vi "RVHR - Configure Language Settings.vi"(7 "Directory Path":path, 8 "error in (no error)":errorcluster, 10 "Supervisory Config Cluster Out":T2={"UI Information"={"Header Image"=path "../Data/header.png", "Language"=enum."English", "First Run?"=FALSE, "Setup Camera?"=FALSE, "Device Type"=enum."RCA", "Encoder Type"=enum."Tacho", "Version"=enum."RailMeasurement_CAT", "port"=0, "greyscale"=FALSE, "camera index"=0}, "Test Cluster"={"Operator"="", "Description"="", "Line"="", "Start Position"=450000.0, "Run Length"=31.0, "Sensor A Position"=80000.0, "Rail Side"=FALSE, "Distance Direction"=FALSE, "Path"=path "", "Sensor B Position"=0.0, "Visible Chart Distance"=0.0, "Company"="", "Ref Profile"=""}, "RV-HR Settings Cluster"={"Sensor A Calibration"=0.0, "Integrator Time"=0.0, "Encoder Spacing"=0.0, "Encoder Threshold"=0.0, "Sampling Distance"=0, "Swap Direction?"=FALSE, "Min Walking Speed"=0.0, "Max Walking Speed"=0.0, "Distance Format"=0, "Sensor B Calibration"=0.0, "Tacho Pulses/Rev"=0.0, "Wheel Diameter"=0.0, "Max Short Roughness"=0.0, "Max Long Roughness"=0.0, "Measuring Interval"=0.0, "Measuring Length"=0.0, "Wavelengths"=[], "Device Resolution"=0, "Detect Change in Direction?"=FALSE, "Save Images?"=FALSE, "Image Frequency"=0, "Save Video?"=FALSE, "Image Offset"=0.0, "Start Position at 0m?"=FALSE, "Live Corrug Est.?"=FALSE, "Wavelength Corrug"=0, "Distance Corrug"=0, "Update Corrug"=0}} {"RV-HR Settings Cluster"."Image Frequency" items=["2", "3", "5"]; "RV-HR Settings Cluster"."Device Resolution" items=["0.1 µm", "1 µm", "10 µm"]; "RV-HR Settings Cluster"."Distance Format" items=["kilometres", "miles & chains", "metres", "stations", "miles"]; "RV-HR Settings Cluster"."Sampling Distance" items=["1mm", "2mm"]}, 11 "UI References":T13) -> (0 "error out":errorcluster, 2 "Language Config Cluster Out":T1={"Home"="Home", "Test Setup"="Setup", "Run Test"="Test", "Configure"="Config", "Hardware Viewer"="Viewer", "Review Test"="Review", "Report"="Home", "Exit"="Exit", "Device Connected?"="Device Connected?", "Test in Progress?"="Test in Progress?", "Simulate?"="Simulate?", "Device Type 1"="Corrugation Analysis Trolley", "Device Type 2"="Bi-Corrugation Analysis Trolley", "Device Type 3"="Bi-Corrugation Analysis Trolley", "Device Type 4"="Bi-Corrugation Analysis Trolley", "Device Type 5"="Bi-Corrugation Analysis Trolley", "Device Type 6"="Bi-Corrugation Analysis Trolley", "Device Type 7"="Bi-Corrugation Analysis Trolley", "Software Version"="Version", "Support"="Software by RailMeasurement Limited - Cambridge - UK - support@railmeasurement.com", "Operator"="Operator:", "Test Description"="Description:", "Line"="Description:", "Test Folder Path"="Folder Path:", "Test Folder Path RCA"="Folder Path:", "Start Position"="Start Position:", "Sensor Position"="Sensor Position:", "Sensor A Position"="Sensor A Position:", "Sensor B Position"="Sensor B Position:", "Visible Chart Distance"="Sensor B Position:", "Rail Side"="Rail Side:", "Rail A Side"="Rail A Side:", "Distance Direction"="Distance Direction:", "Start"="Start:", "Distance Travelled"="Distance Travelled:", "Current Position"="Current Position:", "Stop Test"="Stop", "Pause Test"="Save", "Displacement"="Displacement", "Position"="Position", "Sensor Calibration"="Sensor Calibration:", "Sensor A Calibration"="Sensor A Calibration:", "Sensor B Calibration"="Sensor B Calibration:", "Encoder Spacing"="Encoder Spacing:", "Sampling Distance"="Sampling Distance:", "Tacho Pulses/Rev"="Sensor Calibration:", "Wheel Diameter"="Sensor A Calibration:", "Sampling Distances"=["1mm", "2mm"], "Distance Unit"="Distance in:", "Distance Units"=["Kilometres", "miles & chains", "metres", "stations", "miles"], "Swap Direction"="Swap Direction at Run End?", "Language"="Language", "Device Resolution"="Save", "Device Resolutions"=["Kilometres", "miles & chains", "metres", "stations", "miles"], "Detect Change in Direction"="Save", "Save Config"="Save", "Encoder Data"="Encoder Data", "Sensor Data"="Sensor Data", "Sensor A Data"="Sensor A Data", "Sensor B Data"="Sensor B Data", "Voltage"="Voltage", "Time (m:s)"="Time (m:s)", "Unit mm/s/V"="(mm/s)/V", "Unit mm"="mm", "Unit km"="km", "Unit m"="m", "Start Test Message"="m", "Stop Test Message"="km", "Exit Message"="mm", "File Exists Message"="mm", "File Path Invalid Message"="mm", "Combine Error"="mm", "Combine Success"="mm", "Roller Comp Error"="mm", "Test Folder Path (Live)"="mm", "Folder Error"="Sensor B Position:", "Enc Count"="Setup", "Run Start"="mm", "Run End"="mm", "Date"="mm", "Train"="Sensor B Position:", "Location"="Setup", "Notes"="mm", "Heading_1"="mm", "Heading_2"="mm", "Left Rail"="Sensor B Position:", "Right Rail"="Setup", "Left Exclusions"="mm", "Right Exclusions"="mm", "Settings"="mm", "Wavelength Ranges"="Sensor B Position:", "Y-Axis Limits"="Setup", "Exc Limits"="Sensor B Position:", "Other Settings"="Setup", "Distance/Page"="mm", "Distance/Pages"=["Kilometres", "miles & chains", "metres", "stations", "miles"], "Gridlines"="mm", "Report Tolerance"="mm", "Manual Cut"="Sensor B Position:", "Plot Colour"="Distance in:", "Plot Colours"=["Kilometres", "miles & chains", "metres", "stations", "miles"], "EN Standard"="mm", "RiL Standard"="mm", "Custom Standard"="mm", "Resolution"="Distance in:", "Resolutions"=["Kilometres", "miles & chains", "metres", "stations", "miles"], "Exceedence Header"="mm", "Distance (km)"="mm", "Left (%)"="mm", "Right (%)"="Distance in:", "Page"="Distance in:", "Align"="mm", "Main"="mm", "Comparison"="Distance in:", "Offset"="Distance in:", "From"="Distance in:", "To"="Distance in:", "Of"="Distance in:", "File"="mm", "Load New"="mm", "Load Comparison"="Distance in:", "Discard Comparison"="Distance in:", "Print Current Page"="Distance in:", "Print All Pages"="Distance in:", "Print Exceedence Report"="Distance in:", "Plot Main"="Distance in:", "No Comparison Data to Align"="Distance in:", "Run Load Error"="Distance in:", "Report Load Error"="Distance in:", "Cut"="Distance in:", "Remove"="Distance in:", "Config Settings Unsaved"="Distance in:", "Acquisition Paused"="Distance in:", "Please Select One Option Below"="Distance in:", "RCA is Now Stationary"="Distance in:", "Reporting Setting"="Distance in:", "Main Abbreviated"="Distance in:", "Comparison Abbreviated"="Distance in:", "Exceedence Abbreviated"="Distance in:", "Align Comparison"="Distance in:", "Rail Corrugation Analyser Reporting"="Distance in:", "Show Exc. % in Graph"="Distance in:", "Evaluate Sections <100m"="Distance in:", "Evaluate Sections <0.062mile"="Distance in:", "Section Too Short for Evaluation"="Distance in:", "Language Change Prompt"="Distance in:", "Show All"="Distance in:", "Sections_km"="Distance in:", "Sections_mi"="Distance in:", "Vision"="Distance in:", "Vision Report"="Distance in:", "Vision Display"="Distance in:", "Vision Displays"=["Kilometres", "miles & chains", "metres", "stations", "miles"], "Save Images"="Distance in:", "Image Frequency"="Distance in:", "Section"="Distance in:", "Brightness"="Distance in:", "Contrast"="Distance in:", "Shadow"="Distance in:", "Sharpened"="Distance in:", "Apply to all Images"="Distance in:", "Reset"="Distance in:", "Are you sure"="Distance in:", "Image Processing"="Distance in:", "Save Video"="Distance in:", "Image Offset"="Distance in:", "Camera Mode"="Distance in:", "Camera Modes"=["Kilometres", "miles & chains", "metres", "stations", "miles"], "Copy Page"="Distance in:", "Copy Graphs"="Distance in:", "Camera Mode Change Prompt"="Distance in:", "Camera_1 Missing"="Distance in:", "Camera_2 Missing"="Distance in:", "Cameras Missing"="Distance in:", "Camera Setup"="Distance in:", "Camera_1 Connection Error"="Distance in:", "Camera_2 Connection Error"="Distance in:", "Cameras Connection Error"="Distance in:", "No GPS"="Distance in:", "No Signal"="Distance in:", "Camera_1 Connected"="Distance in:", "Camera_1 Not Connected"="Distance in:", "Camera_2 Connected"="Distance in:", "Camera_2 Not Connected"="Distance in:", "Start Position at 0m?"="Distance in:", "Continue"="Distance in:", "New Test, Same Direction"="Distance in:", "New Test, Opposite Direction"="Distance in:", "Stop and Save"="Distance in:", "Live Corrug Estimate"="Distance in:", "Wavelength Corrug"="Distance in:", "Distance Corrug "="Distance in:", "Update Corrug"="Distance in:", "Company"="Distance in:", "Ref Profile "="Distance in:"})   [LabVIEW 2024]
uses:
  Controls/RVHR - Setting refs.ctl
  Controls/Supervisory Config Cluster.ctl
  Controls/UI Init Config Info.ctl
  Controls/Language.ctl
  Controls/Device_Type.ctl
  Controls/EncoderType.ctl
  Controls/Software Version.ctl
  Controls/Test Cluster.ctl
  Controls/Settings Cluster.ctl
  Controls/Sampling DIstance.ctl
  Controls/Distance Units.ctl
  Controls/Device_Resolution.ctl
  Controls/Language Text Cluster.ctl
  <vilib>/addons/Tools/Unicode/UI Unicode Tools.lvlib
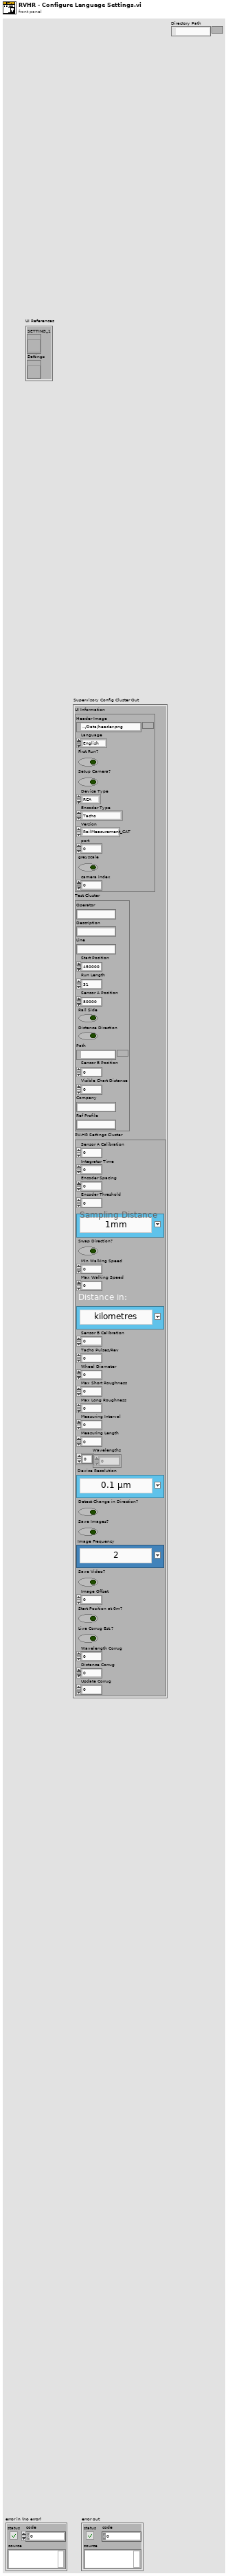
[diagram p1: front panel]
types:
  T1 = typedef "Language Text Cluster.ctl" = cluster{"Home":string, "Test Setup":string, "Run Test":string, "Configure":string, "Hardware Viewer":string, "Review Test":string, "Report":string, "Exit":string, "Device Connected?":string, "Test in Progress?":string, "Simulate?":string, "Device Type 1":string, "Device Type 2":string, "Device Type 3":string, "Device Type 4":string, "Device Type 5":string, "Device Type 6":string, "Device Type 7":string, "Software Version":string, "Support":string, "Operator":string, "Test Description":string, "Line":string, "Test Folder Path":string, "Test Folder Path RCA":string, "Start Position":string, "Sensor Position":string, "Sensor A Position":string, "Sensor B Position":string, "Visible Chart Distance":string, "Rail Side":string, "Rail A Side":string, "Distance Direction":string, "Start":string, "Distance Travelled":string, "Current Position":string, "Stop Test":string, "Pause Test":string, "Displacement":string, "Position":string, "Sensor Calibration":string, "Sensor A Calibration":string, "Sensor B Calibration":string, "Encoder Spacing":string, "Sampling Distance":string, "Tacho Pulses/Rev":string, "Wheel Diameter":string, "Sampling Distances":string[], "Distance Unit":string, "Distance Units":string[], "Swap Direction":string, "Language":string, "Device Resolution":string, "Device Resolutions":string[], "Detect Change in Direction":string, "Save Config":string, "Encoder Data":string, "Sensor Data":string, "Sensor A Data":string, "Sensor B Data":string, "Voltage":string, "Time (m:s)":string, "Unit mm/s/V":string, "Unit mm":string, "Unit km":string, "Unit m":string, "Start Test Message":string, "Stop Test Message":string, "Exit Message":string, "File Exists Message":string, "File Path Invalid Message":string, "Combine Error":string, "Combine Success":string, "Roller Comp Error":string, "Test Folder Path (Live)":string, "Folder Error":string, "Enc Count":string, "Run Start":string, "Run End":string, "Date":string, "Train":string, "Location":string, "Notes":string, "Heading_1":string, "Heading_2":string, "Left Rail":string, "Right Rail":string, "Left Exclusions":string, "Right Exclusions":string, "Settings":string, "Wavelength Ranges":string, "Y-Axis Limits":string, "Exc Limits":string, "Other Settings":string, "Distance/Page":string, "Distance/Pages":string[], "Gridlines":string, "Report Tolerance":string, "Manual Cut":string, "Plot Colour":string, "Plot Colours":string[], "EN Standard":string, "RiL Standard":string, "Custom Standard":string, "Resolution":string, "Resolutions":string[], "Exceedence Header":string, "Distance (km)":string, "Left (%)":string, "Right (%)":string, "Page":string, "Align":string, "Main":string, "Comparison":string, "Offset":string, "From":string, "To":string, "Of":string, "File":string, "Load New":string, "Load Comparison":string, "Discard Comparison":string, "Print Current Page":string, "Print All Pages":string, "Print Exceedence Report":string, "Plot Main":string, "No Comparison Data to Align":string, "Run Load Error":string, "Report Load Error":string, "Cut":string, "Remove":string, "Config Settings Unsaved":string, "Acquisition Paused":string, "Please Select One Option Below":string, "RCA is Now Stationary":string, "Reporting Setting":string, "Main Abbreviated":string, "Comparison Abbreviated":string, "Exceedence Abbreviated":string, "Align Comparison":string, "Rail Corrugation Analyser Reporting":string, "Show Exc. % in Graph":string, "Evaluate Sections <100m":string, "Evaluate Sections <0.062mile":string, "Section Too Short for Evaluation":string, "Language Change Prompt":string, "Show All":string, "Sections_km":string, "Sections_mi":string, "Vision":string, "Vision Report":string, "Vision Display":string, "Vision Displays":string[], "Save Images":string, "Image Frequency":string, "Section":string, "Brightness":string, "Contrast":string, "Shadow":string, "Sharpened":string, "Apply to all Images":string, "Reset":string, "Are you sure":string, "Image Processing":string, "Save Video":string, "Image Offset":string, "Camera Mode":string, "Camera Modes":string[], "Copy Page":string, "Copy Graphs":string, "Camera Mode Change Prompt":string, "Camera_1 Missing":string, "Camera_2 Missing":string, "Cameras Missing":string, "Camera Setup":string, "Camera_1 Connection Error":string, "Camera_2 Connection Error":string, "Cameras Connection Error":string, "No GPS":string, "No Signal":string, "Camera_1 Connected":string, "Camera_1 Not Connected":string, "Camera_2 Connected":string, "Camera_2 Not Connected":string, "Start Position at 0m?":string, "Continue":string, "New Test, Same Direction":string, "New Test, Opposite Direction":string, "Stop and Save":string, "Live Corrug Estimate":string, "Wavelength Corrug":string, "Distance Corrug ":string, "Update Corrug":string, "Company":string, "Ref Profile ":string}
  T2 = typedef "Supervisory Config Cluster.ctl" = cluster{"UI Information":T3, "Test Cluster":T8, "RV-HR Settings Cluster":T9}
  T3 = typedef "UI Init Config Info.ctl" = cluster{"Header Image":path, "Language":T4, "First Run?":bool, "Setup Camera?":bool, "Device Type":T5, "Encoder Type":T6, "Version":T7, "port":i32, "greyscale":bool, "camera index":i32}
  T4 = typedef "Language.ctl" = enum16{"English", "Chinese", "German"}
  T5 = typedef "Device_Type.ctl" = enum16{"CAT", "Bi-CAT", "YRCA", "RCA", "RV-HR", "TV-HR"}
  T6 = typedef "EncoderType.ctl" = enum16{"Tacho", "Quadrature"}
  T7 = typedef "Software Version.ctl" = enum16{"RailMeasurement_CAT", "RailMeasurement_Master", "RailMeasurement_RCA", "RailMeasurement_CAT-V", "RailMeasurement_RCA-V", "RailMeasurement_RV-HR"}
  T8 = typedef "Test Cluster.ctl" = cluster{"Operator":string, "Description":string, "Line":string, "Start Position":dbl, "Run Length":dbl, "Sensor A Position":dbl, "Rail Side":bool, "Distance Direction":bool, "Path":path, "Sensor B Position":dbl, "Visible Chart Distance":dbl, "Company":string, "Ref Profile":string}
  T9 = typedef "Settings Cluster.ctl" = cluster{"Sensor A Calibration":dbl, "Integrator Time":dbl, "Encoder Spacing":dbl, "Encoder Threshold":dbl, "Sampling Distance":T10, "Swap Direction?":bool, "Min Walking Speed":dbl, "Max Walking Speed":dbl, "Distance Format":T11, "Sensor B Calibration":dbl, "Tacho Pulses/Rev":dbl, "Wheel Diameter":dbl, "Max Short Roughness":dbl, "Max Long Roughness":dbl, "Measuring Interval":dbl, "Measuring Length":dbl, "Wavelengths":dbl[], "Device Resolution":T12, "Detect Change in Direction?":bool, "Save Images?":bool, "Image Frequency":T10, "Save Video?":bool, "Image Offset":dbl, "Start Position at 0m?":bool, "Live Corrug Est.?":bool, "Wavelength Corrug":u8, "Distance Corrug":u8, "Update Corrug":u8}
  T10 = typedef "Sampling DIstance.ctl" = u16
  T11 = typedef "Distance Units.ctl" = u16
  T12 = typedef "Device_Resolution.ctl" = u16
  T13 = typedef "RVHR - Setting refs.ctl" = cluster{"SETTING_1":refnum<vi>, "Settings":refnum<vi>}
  T14 = typedef "Settings UI Refs.ctl" = cluster{"10-30mm":refnum<vi>, "30-100mm":refnum<vi>, "100-300mm":refnum<vi>, "300-1000mm":refnum<vi>, "Y 10-30mm":refnum<vi>, "Y 30-100mm":refnum<vi>, "Y 100-300mm":refnum<vi>, "Y 300-1000mm":refnum<vi>, "Ex 10-30mm":refnum<vi>, "Ex 30-100mm":refnum<vi>, "Ex 100-300mm":refnum<vi>, "Ex 300-1000mm":refnum<vi>, "Exceedance Resolution":refnum<vi>, "EN13231?":refnum<vi>, "Ril?":refnum<vi>, "Custom?":refnum<vi>, "Distance Per Page":refnum<vi>, "Distance Per Page (Miles)":refnum<vi>, "Exc Limit":refnum<vi>, "Gridlines?":refnum<vi>, "Manual Cut?":refnum<vi>, "Plot Colours":refnum<vi>, "Wavelength Ranges":refnum<vi>, "Y-Axis Limits":refnum<vi>, "Exc Limits":refnum<vi>, "Settings":refnum<vi>}
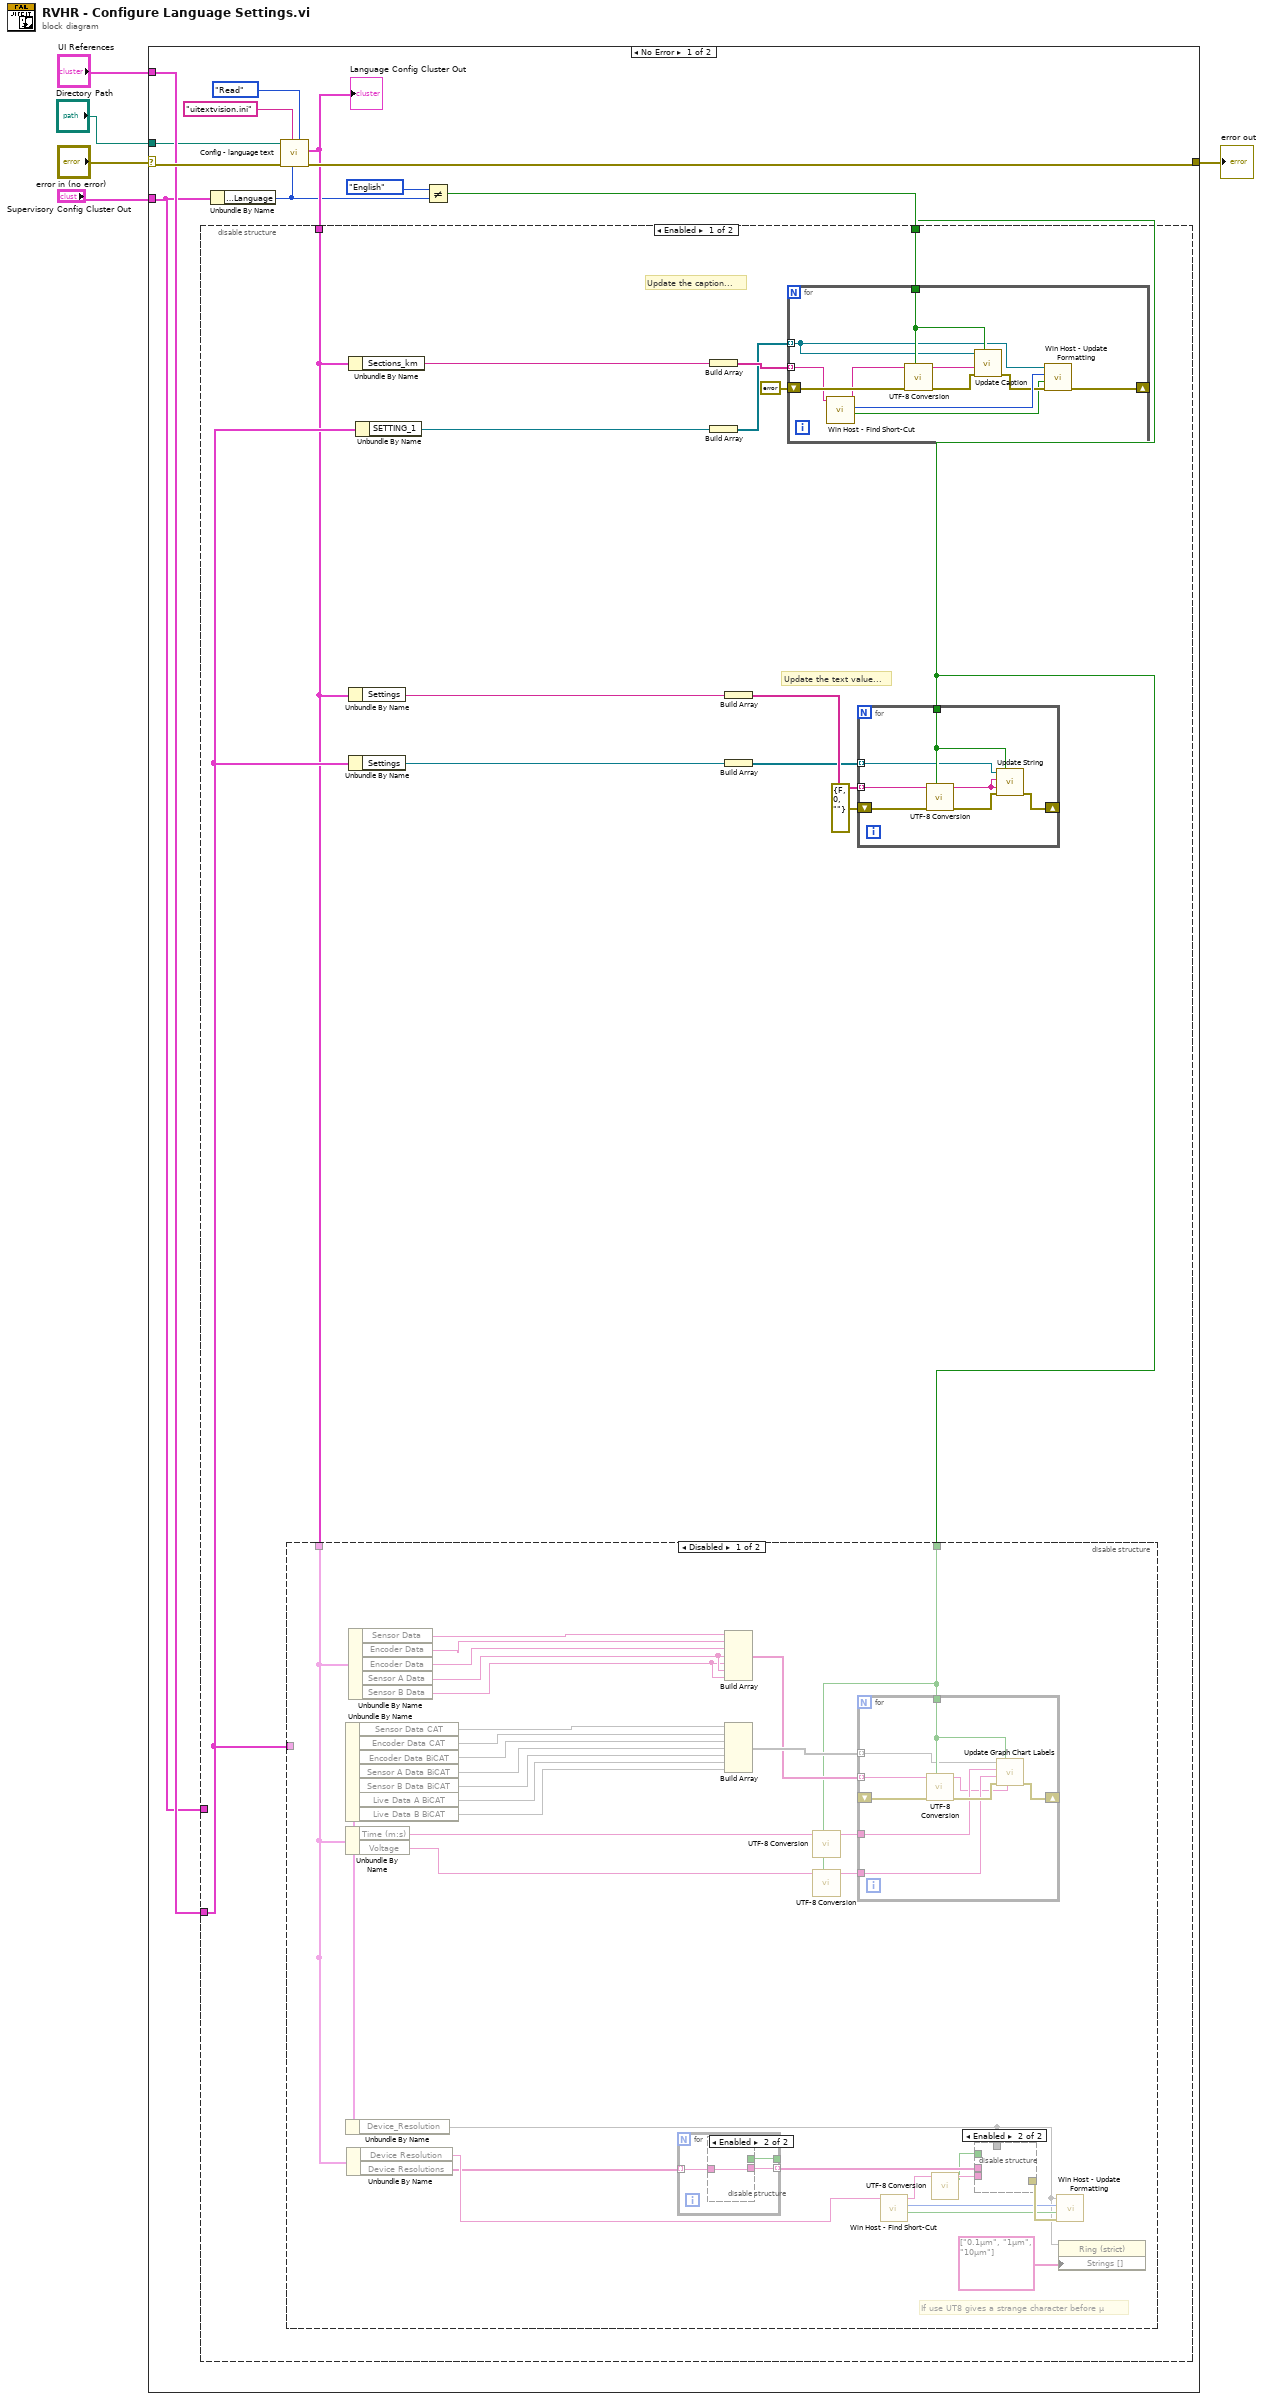
[diagram p0: block diagram]
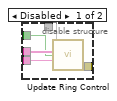
[diagram p2: hidden frame]
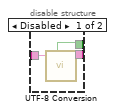
[diagram p3: hidden frame]
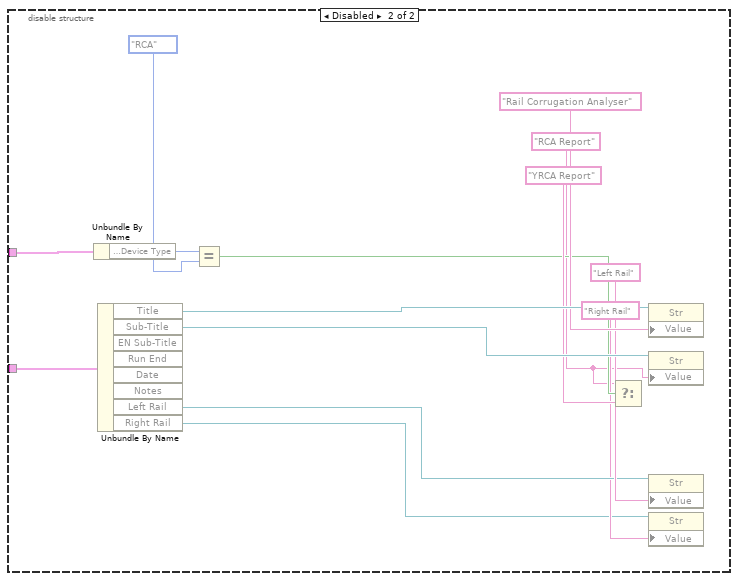
[diagram p5: hidden frame]
diagram:
  n1 = case shown="No Error" "error in (no error)" {
    selector: "error in (no error)" -> [w16 w115]
    tunnel: [w15 w115] -> w4
    tunnel: "UI References" -> [w11 _]
    tunnel: "Supervisory Config Cluster Out" -> [w8 _]
    tunnel: "Directory Path" -> [w9 _]
    frame No Error {
      n2 = Unbundle By Name(w8) -> ("UI Information.Language"=w6:T4)
      n3 = call "Config - language text.vi"(".ini Controller"=enum16{"Read", "Write"}."Read", "Language"=w6, ".ini filename"="uitextvision.ini", "error in (no error)"=w16, "Directory Path"=w9) -> ("error out"=w15:errorcluster, "Language Config Cluster Out"=w10:T1)  [unwired: 4 in, 1 out]
      "Language Config Cluster Out" <- w10
      n4 = Not Equal?(x=Language."English" ("UI Information.Language"), y=w6) -> (x != y?=w7:bool)
      n5 = disable-structure shown="Enabled" {
        disable-tunnel: w11 -> [w27 w101]
        disable-tunnel: w10 -> [w26 _]
        disable-tunnel: w7 -> [w19 _]
        disable-tunnel: w8 -> [_ w110]
        frame Enabled {
          # "Update the text value..."
          # "Update the caption..."
          n6 = disable-structure shown="Disabled" {
            disable-tunnel: w27 -> [_ _]
            disable-tunnel: w26 -> [w54 _]
            disable-tunnel: w19 -> [w53 _]
            frame Disabled {
              # "If use UT8 gives a strange character before µ"
              n7 = Unbundle By Name() -> (w55:T14, "Sensor Data CAT"=w76, "Encoder Data CAT"=w75, "Encoder Data BiCAT"=w74, "Sensor A Data BiCAT"=w73, "Sensor B Data BiCAT"=w72, "Live Data A BiCAT"=w65, "Live Data B BiCAT"=w64)
              n8 = Unbundle By Name(w54) -> ("Time (m:s)"=w69:string, "Voltage"=w68:string)
              n9 = Unbundle By Name(w55) -> ("Device_Resolution"=w51)
              n10 = Unbundle By Name(w54) -> ("Device Resolution"=w52:string, "Device Resolutions"=w50:string[])
              n11 = Unbundle By Name(w54) -> ("Sensor Data"=w79:string, "Encoder Data"=w78:string, "Encoder Data"=w77:string, "Sensor A Data"=w63:string, "Sensor B Data"=w62:string)
              n12 = for {
                tunnel: w50 -> [w87] mode=indexing
                tunnel: _ -> [w86]
                tunnel: [w85] -> w56 mode=indexing
                n13 = disable-structure shown="Enabled" {
                  disable-tunnel: w87 -> [w90 w91]
                  disable-tunnel: w86 -> [w89 _]
                  disable-tunnel: [w88 w91] -> w85
                  frame Disabled {
                    n14 = call "UTF-8 Conversion.vi"("Unicode?"=w89, "Config String"=w90) -> ("Unicode/ANSI string"=w88:string)  [unwired: 8 in, 1 out]
                  }
                  frame Enabled {
                  }
                }
              }
              n15 = Build Array(w79, w78, w77, w63, w62, w63, w62) -> (w70:string[])
              n16 = Build Array(w76, w75, w74, w73, w72, w65, w64) -> (w71:void[])
              n17 = call "UTF-8 Conversion.vi"("Unicode?"=w53, "Config String"=w69) -> ("Unicode/ANSI string"=w67:string)  [unwired: 8 in, 1 out]
              n18 = call "UTF-8 Conversion.vi"("Unicode?"=w53, "Config String"=w68) -> ("Unicode/ANSI string"=w66:string)  [unwired: 8 in, 1 out]
              n19 = for {
                tunnel: w70 -> [w93] mode=indexing
                tunnel: w53 -> [w97]
                tunnel: w71 -> [w96] mode=indexing
                shift-right: [w98] -> _
                shift-left: _ -> [w100]
                tunnel: w67 -> [w95]
                tunnel: w66 -> [w94]
                n20 = call "UTF-8 Conversion.vi"("Unicode?"=w97, "error in"=w100, "Config String"=w93) -> ("error out"=w99:errorcluster, "Unicode/ANSI string"=w92:string)  [unwired: 7 in]
                n21 = call <vilib>:"Update Graph Chart Labels.vi"("Caption"=w92, "Interpret as Unicode (T)"=w97, "error in (no error)"=w99, "Y Axis Label"=w94, "X Axis Label"=w95, "GrphChrt Ref"=w96) -> ("error out"=w98:errorcluster)  [unwired: 4 in, 1 out]
              }
              n22 = call "Win Host - Find Short-Cut.vi"("Language in"=w52) -> ("Short-Cut?"=w59:bool, "S/CUT Index"=w58:i32, "Language out"=w60:string)  [unwired: 8 in]
              n23 = call "UTF-8 Conversion.vi"("Config String"=w60) -> ("Unicode/ANSI string"=w57:string, "Unicode?"=w48:bool)  [unwired: 8 in, 1 out]
              n24 = disable-structure shown="Enabled" {
                disable-tunnel: [w84 _] -> w61
                disable-tunnel: w57 -> [w83 _]
                disable-tunnel: w56 -> [w82 _]
                disable-tunnel: w51 -> [w81 _]
                disable-tunnel: w48 -> [w80 _]
                frame Disabled {
                  n25 = call <vilib>:"Update Ring Control.vi"("Interpret as Unicode (T)"=w80, "Caption"=w83, "Strings"=w82, "Ring Control Ref"=w81) -> ("error out"=w84:errorcluster)  [unwired: 5 in]
                }
                frame Enabled {
                }
              }
              n26 = call "Win Host - Update Formatting.vi"("error in (no error)"=w61, "Short-Cut?"=w59, "Index"=w58, "Control in"=w51) -> ()  [unwired: 7 in, 1 out]
              n27 = property class="Ring (strict)"(reference=w51, "Strings []"=string[] ["0.1µm", "1µm", "10µm"]) -> ()  [unwired: 1 in, 2 out]
            }
            frame Enabled {
            }
          }
          n28 = Unbundle By Name(w26) -> ("Sections_km"=w24:string)
          n29 = Unbundle By Name(w26) -> ("Settings"=w18:string)
          n30 = Unbundle By Name(w27) -> ("Settings"=w17:refnum<vi>)
          n31 = Unbundle By Name(w27) -> ("SETTING_1"=w25:refnum<vi>)
          n32 = Build Array(w24) -> (w29:string[])
          n33 = Build Array(w25) -> (w28:refnum<vi>[])
          n34 = Build Array(w18) -> (w23:string[])
          n35 = Build Array(w17) -> (w22:refnum<vi>[])
          n36 = for {
            tunnel: w29 -> [w36] mode=indexing
            tunnel: w19 -> [w39]
            tunnel: w28 -> [w33] mode=indexing
            shift-right: [w31] -> _
            shift-left: errorcluster {"status"=FALSE, "code"=0, "source"=""} ("error out") -> [w37]
            n37 = call "Win Host - Find Short-Cut.vi"("Language in"=w36) -> ("Short-Cut?"=w30:bool, "S/CUT Index"=w34:i32, "Language out"=w35:string)  [unwired: 8 in]
            n38 = call "UTF-8 Conversion.vi"("Unicode?"=w39, "error in"=w37, "Config String"=w35) -> ("error out"=w38:errorcluster, "Unicode/ANSI string"=w40:string)  [unwired: 7 in]
            n39 = call <vilib>:"Update Caption.vi"("Interpret as Unicode (T)"=w39, "error in (no error)"=w38, "Caption"=w40, "Control Reference"=w33) -> ("error out"=w32:errorcluster)  [unwired: 4 in, 1 out]
            n40 = call "Win Host - Update Formatting.vi"("error in (no error)"=w32, "Short-Cut?"=w30, "Index"=w34, "Control in"=w33) -> ("error out"=w31:errorcluster)  [unwired: 7 in]
          }
          n41 = for {
            tunnel: w23 -> [w42] mode=indexing
            tunnel: w19 -> [w44]
            tunnel: w22 -> [w43] mode=indexing
            shift-right: [w45] -> _
            shift-left: errorcluster {"status"=FALSE, "code"=0, "source"=""} ("error out") -> [w47]
            n42 = call "UTF-8 Conversion.vi"("Unicode?"=w44, "error in"=w47, "Config String"=w42) -> ("error out"=w46:errorcluster, "Unicode/ANSI string"=w41:string)  [unwired: 7 in]
            n43 = call <vilib>:"Update String.vi"("Interpret as Unicode (T)"=w44, "error in (no error)"=w46, "Caption"=w41, "String Value"=w41, "String Control Reference"=w43) -> ("error out"=w45:errorcluster)  [unwired: 3 in, 1 out]
          }
        }
        frame Disabled {
          w102 = "RCA Report" ("Value")
          n44 = Unbundle By Name(w110) -> ("UI Information.Device Type"=w109:T5)
          n45 = Unbundle By Name(w101) -> ("Title"=w114:refnum<vi>, "Sub-Title"=w112:refnum<vi>, "Left Rail"=w105:refnum<vi>, "Right Rail"=w103:refnum<vi>)  [unwired: 4 out]
          n46 = Equal?(x=w109, y=Device_Type."RCA") -> (x = y?=w107:bool)
          n47 = Select(t=w102, s=w107, f="YRCA Report" ("Value")) -> ()  [unwired: 1 out]
          n48 = property class="Str"(reference=w114, "Value"="Rail Corrugation Analyser") -> ()  [unwired: 1 in, 2 out]
          n49 = property class="Str"(reference=w112, "Value"=w102) -> ()  [unwired: 1 in, 2 out]
          n50 = property class="Str"(reference=w105, "Value"="Left Rail") -> ()  [unwired: 1 in, 2 out]
          n51 = property class="Str"(reference=w103, "Value"="Right Rail") -> ()  [unwired: 1 in, 2 out]
        }
      }
    }
    frame Error {
    }
  }
  "error out" <- w4
